vi "PH_PSDBController.constructor.vi"(0 "name":string, 2 "data in":string, 5 "error in":errorcluster) -> (14 "i ref out":refnum<vi>, 16 "data out":string, 19 "error out":errorcluster)   [LabVIEW 2014, in "PH_PSDBController.lvlib"]
doc: "This class is forseen to collect data of PHELIX devices around a PHELIX shot. It uses the ReadData-Method and stores the data in LabVIEW format. They can be visualized using the class PH_DataViewer. \n\nThis class is part of the PHELIX application layer.\n\nauthor: Stefan Götte, GSI\n\nLicense Agreement for this software:\n\nCopyright (C)\nGesellschaft für Schwerionenforschung, GSI\nPlanckstr. 1\n64291 Darmstadt\nGermany\n\nContact: D.Beck@gsi.de \n\nThis program is free software; you can redistribute it and/or modify it under the terms of the \nGNU General Public License as published by the Free Software Foundation; either version 2 of \nthe license, or (at your option) any later version.\n\nThis program is distributed in the hope that it will be useful, but WITHOUT ANY WARRANTY; \nwithout even the implied warranty of MERCHANTABILITY or FITNESS FOR A PARTICULAR PURPOSE. See the GNU General License for more details (http://www.gnu.org).\n\nGesellschaft für Schwerionenforschung, GSI\nPlanckstr. 1, 64291 Darmstadt, Germany\nFor all questions and ideas contact: M.Richter@gsi.de, H.Brand@gsi.de or D.Beck@gsi.de.\nLast update: 16-JUN-2004"
uses:
  PH_PSDBController.lvlib
  CS_Core/CSObj/CSObj.lvlib
  PH_Basics/PH_Class/PH_Class.lvlib
  PH_Basics/PH_StatusHandler/PH_StatusHandler.lvlib
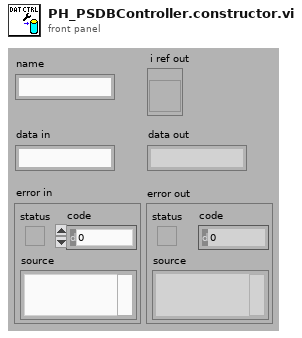
[diagram p1: front panel]
types:
  T1 = enum16{"SetAttribute", "GetAttribute", "CreateAttribute", "DestroyAttribute", "DestroyAllAtributes"}
  T2 = typedef "PH_PSDBController.lvlib/PH_PSDBController.i attribute.ctl" = cluster{"GUI Refs":cluster{"Data Status":refnum<vi>, "Current Shot ID":refnum<vi>, "active Subsystems":refnum<vi>, "Experiment Description":refnum<vi>, "Shot Comment":refnum<vi>, "Experiment":refnum<vi>, "Shottype":refnum<vi>, "Sequencer SM State":refnum<vi>, "Instances with Errors":refnum<vi>}, "Service ID Shot ID":i32, "Service ID wanted Subsystem":i32, "Data Status":T3, "Shotinformation":cluster{"Current Experiment ID":i32, "Current Shot Type":i32, "Current Comment":string}, "Data taking?":bool, "Service ID current Shottype":i32, "Service ID current Experiment":i32, "Service ID currentShot Comment":i32, "Service ID possible Shottypes":i32, "Service ID possible Experiments":i32, "possible Experiments":T4[], "possible Shottypes":T4[], "List":cluster{"Info":cluster{"Instance":string, "Data Status":T3}[], "GUI Ref":refnum<vi>, "Classname":string}[], "Subsystems Off?":cluster{"PHELIX_Beamline_fs_YLF_BL_Status":bool, "PHELIX_Beamline_ns_BL_Status":bool, "PHELIX_Beamline_PA_Input_BL_Status":bool, "PHELIX_Beamline_PA_MA_BL_Status":bool, "PHELIX_Beamline_MA_Z6_BL_Status":bool, "PHELIX_Beamline_MA_LB_BL_Status":bool, "PHELIX_Beamline_PA_LL_BL_Status":bool}, "PSDB Credentials":T5}
  T3 = typedef "PH_PSDBWriter.lvlib/PH_PSDBWriter.Data Status.ctl" = i16
  T4 = typedef "PSDB.lvlib/PSDB_Info.ctl" = cluster{"Name":string, "Description":string, "ID":i32}
  T5 = typedef "PH_Common.lvlib/PH_Connection.PSDB Credentials.ctl" = cluster{"PW":string, "ID":string, "DS":string}
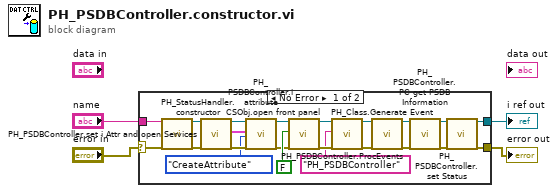
[diagram p0: block diagram]
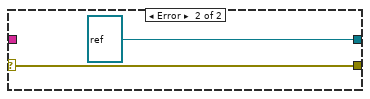
[diagram p2: hidden frame]
diagram:
  n1 = case shown="No Error" "error in" {
    selector: "error in" -> [w26 w28]
    tunnel: [w21 refnum<vi> refnum ("i ref out")] -> w4
    tunnel: [w20 w28] -> w3
    tunnel: "name" -> [w25 _]
    frame No Error {
      n2 = call "PH_StatusHandler.constructor.vi"("name"=w25, "error in(no error)"=w26) -> ("i ref out"=w13:refnum<vi>, "error out"=w14:errorcluster)  [unwired: 15 in, 1 out]
      n3 = call "PH_PSDBController.set i Attr and open Services.vi"("i ref in"=w13, "error in"=w14) -> ("i ref out"=w12:refnum<vi>, "i Attributes"=w10:T2, "error out"=w11:errorcluster)  [unwired: 15 in]
      n4 = call "PH_PSDBController.i attribute.vi"("VI Refnum"=w12, "CLASS.i attribute"=w10, "Action"=T1."CreateAttribute", "error in (no error)"=w11) -> ("VI Refnum out"=w6:refnum<vi>, "error out"=w7:errorcluster)  [unwired: 13 in, 1 out]
      n5 = call "CSObj.open front panel.vi"("i ref in"=w6, "frontPanelOpen"=FALSE ("front panel open"), "error in (no error)"=w7) -> ("i ref out"=w23:refnum<vi>, "error out"=w22:errorcluster)  [unwired: 15 in]
      n6 = call "PH_Class.Generate Event.vi"("i ref in"=w23, "Class"="PH_PSDBController", "error in (no error)"=w22) -> ("i ref out"=w8:refnum<vi>, "error out"=w15:errorcluster)  [unwired: 15 in]
      n7 = call "PH_PSDBController.ProcEvents.vi"("i ref in"=w8, "error in"=w15) -> ("i ref out"=w17:refnum<vi>, "error out"=w19:errorcluster)  [unwired: 16 in]
      n8 = call "PH_PSDBController.PC get PSDB Information.vi"("i ref in"=w17, "error IO"=w19) -> ("i ref out"=w16:refnum<vi>, "error out"=w18:errorcluster)  [unwired: 16 in]
      n9 = call "PH_PSDBController.set Status.vi"("i ref in"=w16, "error in"=w18) -> ("i ref out"=w21:refnum<vi>, "error out"=w20:errorcluster)  [unwired: 16 in]
    }
    frame Error {
    }
  }
  "i ref out" <- w4
  "error out" <- w3
